vi "Open Client Connection.vi"(8 "error in (no error)":errorcluster, 9 "Port":u16, 10 "address":string, 11 "RemoteControl in":refnum<class "RemoteControl.lvclass">) -> (0 "error out":errorcluster, 3 "RemoteControl out":refnum<class "RemoteControl.lvclass">)   [LabVIEW 2019, in "RemoteControl.lvlib" / "RemoteControl.lvclass"]
uses:
  RemoteControl.lvclass
  Typedefs/RC Process Type--Enum.ctl
  RemoteControl.lvclass/RemoteControl.ctl
  Private/RemoteControl.GlobalVariable.vi
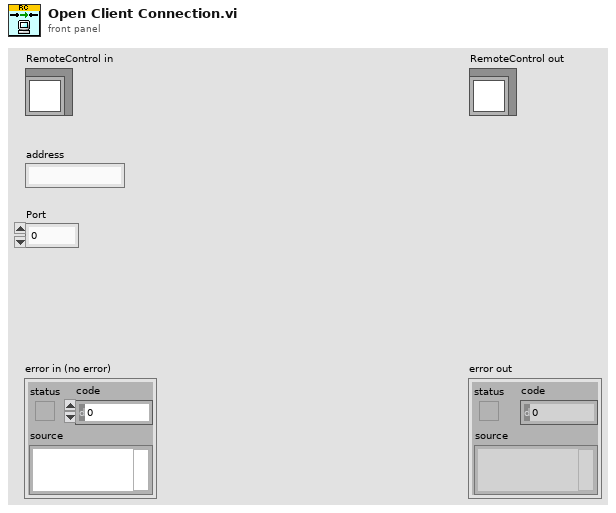
[diagram p1: front panel]
types:
  T1 = typedef "RemoteControl.lvlib/RemoteControl.lvclass/RC Process Type--Enum.ctl" = enum16{"Listener", "Server", "Client"}
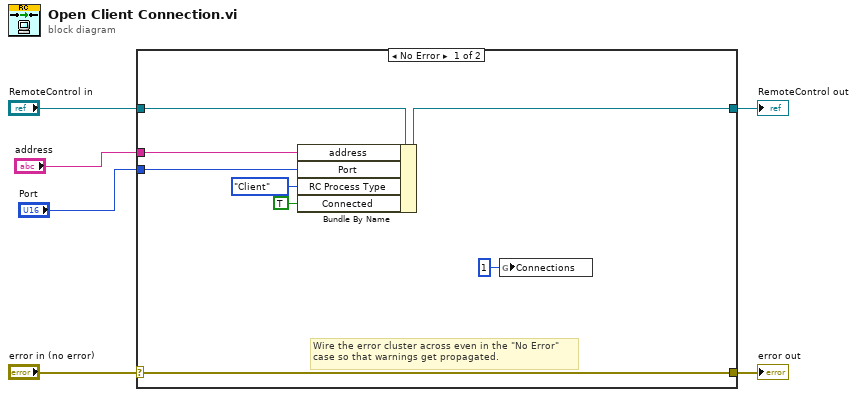
[diagram p0: block diagram]
diagram:
  n1 = case shown="No Error" "error in (no error)" {
    selector: "error in (no error)" -> [w14 w16]
    tunnel: [w14 w16] -> w5
    tunnel: [w12 w15] -> w3
    tunnel: "RemoteControl in" -> [w13 w15]
    tunnel: "Port" -> [w11 _]
    tunnel: "address" -> [w10 _]
    frame No Error {
      # "Wire the error cluster across even in the \"No Error\"\ncase so that warnings get propagated."
      n2 = Bundle By Name(cluster=w13, "address"=w10, "Port"=w11, "RC Process Type"=RC_Process_Type--Enum."Client", "Connected"=TRUE ("Created")) -> (w12:refnum<class "RemoteControl.lvclass">)
      n3 = global write "RemoteControl.GlobalVariable.vi" "Connections"(1 ("Connections")) -> ()
    }
    frame Error {
    }
  }
  "error out" <- w5
  "RemoteControl out" <- w3
